vi "Compare.vi"(8 "error in (no error)":errorcluster, 10 "fpMgr in":refnum<class "VIProviderShellHelper.lvclass">, 11 "Shell in":refnum<class "VIProviderShellHelper.lvclass">) -> (0 "error out":errorcluster, 1 "Matched":bool, 2 "fpMgr out":refnum<class "VIProviderShellHelper.lvclass">, 3 "Shell out":refnum<class "VIProviderShellHelper.lvclass">)   [LabVIEW 2019, in "LabVIEW-VIProviderShell.lvlib" / "VIProviderShellHelper.lvclass"]
uses:
  VIProviderShellHelper.lvclass
  VIProviderShellHelper.lvclass/VIProviderShellHelper.ctl
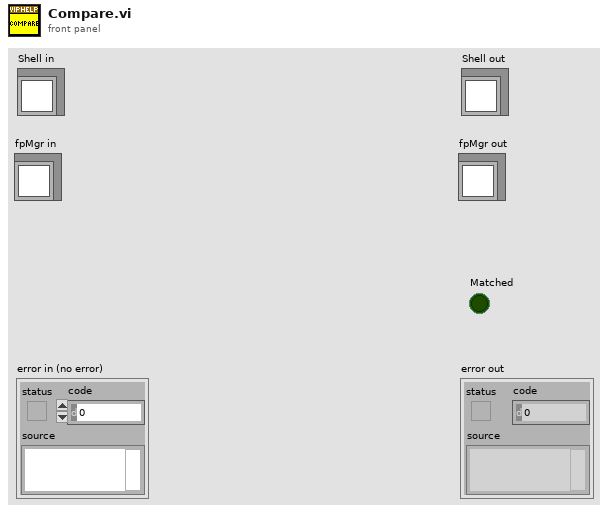
[diagram p1: front panel]
types:
  T1 = typedef "LabVIEW-VIProviderShell.lvlib/VIProviderShellHelper.lvclass/def-ConnectorInfo.ctl" = cluster{"Value":variant, "Label.Text":string, "error":errorcluster, "DatatypeDescription":string, "Indicator":bool}
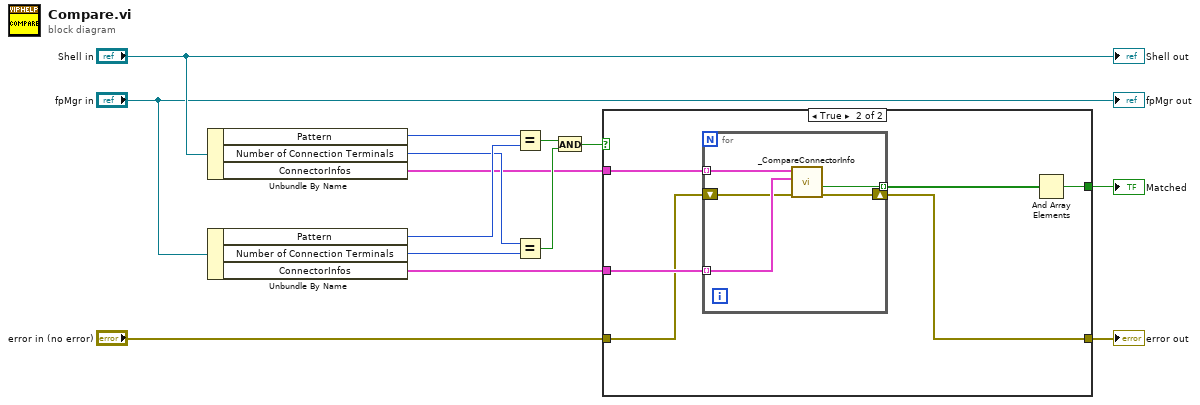
[diagram p0: block diagram]
diagram:
  n1 = Unbundle By Name("Shell in") -> ("Pattern"=w12:u32, "Number of Connection Terminals"=w10:u32, "ConnectorInfos"=w2:T1[])
  n2 = Unbundle By Name("fpMgr in") -> ("Pattern"=w11:u32, "Number of Connection Terminals"=w9:u32, "ConnectorInfos"=w1:T1[])
  n3 = Equal?(x=w12, y=w11) -> (x = y?=w8:bool)
  n4 = Equal?(x=w10, y=w9) -> (x = y?=w7:bool)
  n5 = And(x=w8, y=w7) -> (x .and. y?=w6:bool)
  n6 = case shown="True" w6 {
    tunnel: w2 -> [_ w21]
    tunnel: w1 -> [_ w20]
    tunnel: [_ w19] -> w5
    tunnel: "error in (no error)" -> [w15 w17]
    tunnel: [w15 w16] -> w3
    frame False {
    }
    frame True {
      n7 = for {
        tunnel: w21 -> [w26] mode=indexing
        tunnel: w20 -> [w25] mode=indexing
        tunnel: [w24] -> w18 mode=indexing
        shift-right: [w22] -> w16
        shift-left: w17 -> [w23]
        n8 = call "_CompareConnectorInfo.vi"("error in (no error)"=w23, 10:"Cluster"=w25, 11:"Cluster"=w26) -> ("error out"=w22:errorcluster, "Matched"=w24:bool)  [unwired: 5 in, 2 out]
      }
      n9 = And Array Elements(Boolean array=w18) -> (logical AND=w19:bool)
    }
  }
  "error out" <- w3
  "Matched" <- w5
  "Shell out" <- "Shell in"
  "fpMgr out" <- "fpMgr in"
